vi "ApplicationTemplate.vi"() -> ()   [LabVIEW 2020]
uses:
  VI Server Toolkit/VI Server Toolkit LV2013.lvlib
panel:
  in  "Stop":bool
  out "error out":errorcluster
  in  "error in (no error)":errorcluster
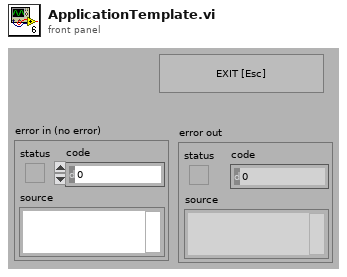
[diagram p1: front panel]
types:
  T1 = typedef "Labels&Control References.ctl" = cluster{"Refs":refnum<vi>[], "Labels":string[], "VI Ref":refnum<vi>}
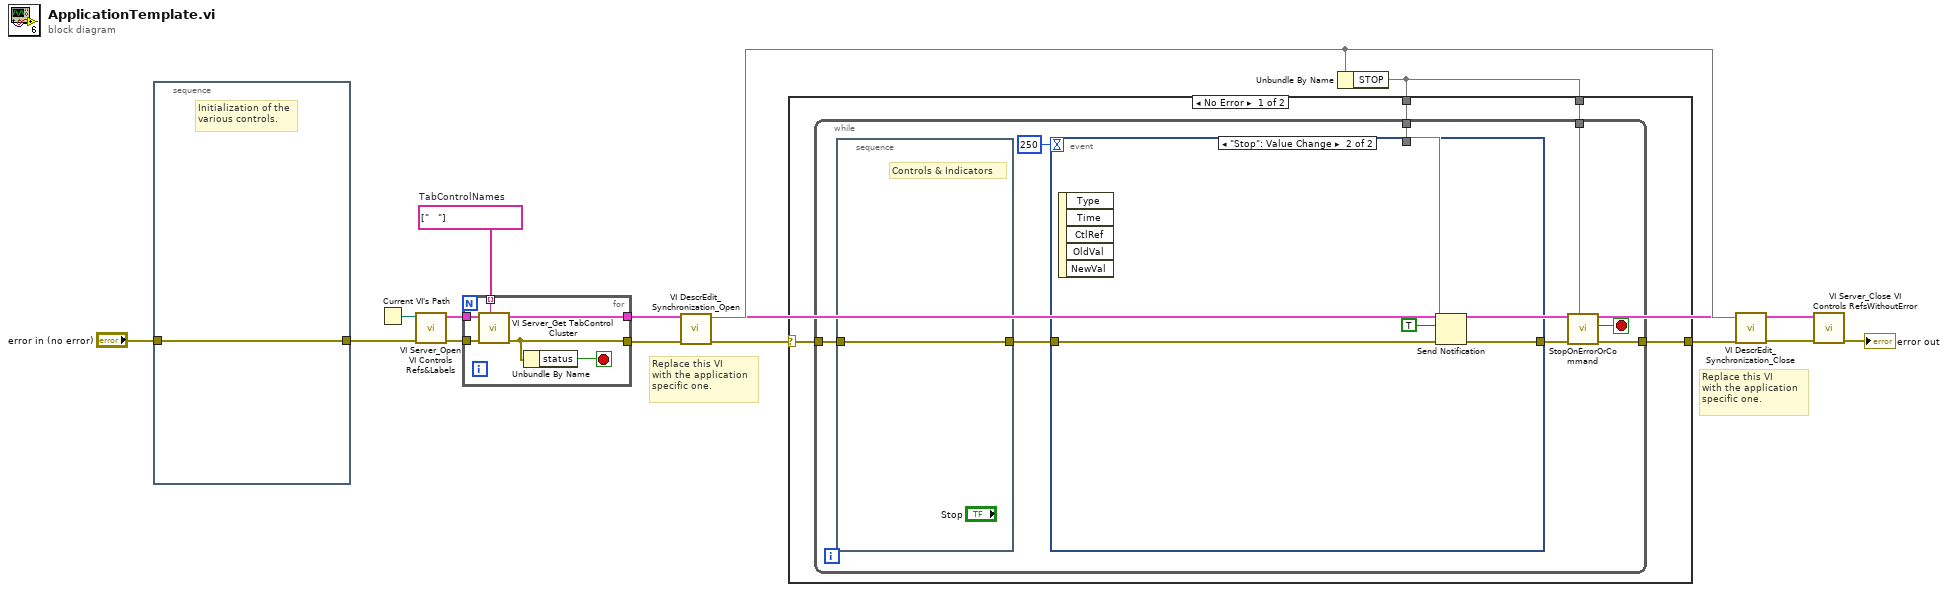
[diagram p0: block diagram]
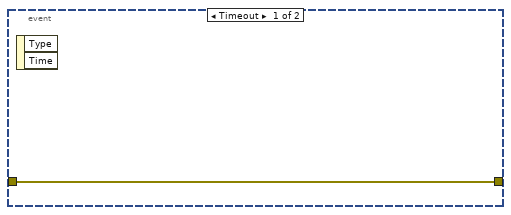
[diagram p2: hidden frame]
diagram:
  w9 = string[] ["   "]  # TabControlNames
  # "Replace this VI\nwith the application\nspecific one."
  # "Replace this VI\nwith the application\nspecific one."
  n1 = stacked-sequence {
    tunnel: "error in (no error)" -> [w15]
    tunnel: [w15] -> w13
    frame #0 {
      # "Initialization of the\nvarious controls."
    }
  }
  n2 = Current VI's Path() -> (path=w12:path)
  n3 = call "VI Server_Open VI Controls Refs&Labels.vi"("error in (no error)"=w13, "vi path"=w12) -> ("error out"=w11:errorcluster, "Labels&Refs"=w10:T1)  [unwired: 8 in]
  n4 = for {
    tunnel: w11 -> [w21]
    tunnel: w10 -> [w20]
    tunnel: [w17] -> w8
    tunnel: [w19] -> w2
    tunnel: w9 -> [w18] mode=indexing
    stop <- w16 stop-if-true
    n5 = call "VI Server_Get TabControl Cluster.vi"("TabControl Label"=w18, "error in"=w21, "VI Server Cluster.IN"=w20) -> ("error out"=w17:errorcluster, "VI Server Cluster.OUT"=w19:T1)  [unwired: 7 in]
    n6 = Unbundle By Name(w17) -> ("status"=w16:bool)
  }
  n7 = call "VI DescrEdit_Synchronization_Open.vi"("error in (no error)"=w8) -> ("error out"=w7:errorcluster, 3:w5)  [unwired: 9 in]
  n8 = Unbundle By Name(w5) -> ("STOP"=w4)
  n9 = case shown="No Error" w7 {
    selector: w7 -> [w25 w40]
    tunnel: [w24 w40] -> w6
    tunnel: w4 -> [w23 _]
    tunnel: w4 -> [w22 _]
    frame No Error {
      n10 = while {
        tunnel: w25 -> [w33]
        tunnel: [w30] -> w24
        tunnel: w23 -> [w28]
        tunnel: w22 -> [w26]
        stop <- w27 stop-if-true
        n11 = stacked-sequence {
          tunnel: w33 -> [w39]
          tunnel: [w39] -> w31
          frame #0 {
            # "Controls & Indicators"
          }
        }
        n12 = event shown="[1] \"Stop\": Value Change" {
          selector: _ -> [_ _]
          dyn-events: _ -> [_ _]
          timeout: 250 -> [_ _]
          tunnel: w31 -> [w34 w38]
          tunnel: [w34 w37] -> w29
          tunnel: w26 -> [_ w36]
          event Timeout {
            n13 = event-data() -> ()  [unwired: 1 in, 2 out]
          }
          event "Stop": Value Change {
            n14 = event-data() -> ()  [unwired: 1 in, 5 out]
            n15 = Send Notification(notification=TRUE, notifier=w36, error in (no error)=w38) -> (error out=w37:errorcluster)  [unwired: 1 out]
          }
        }
        n16 = call "StopOnErrorOrCommand.vi"("STOP"=w28, "error in (no error)"=w29) -> ("error out"=w30:errorcluster, "STOP"=w27:bool)  [unwired: 8 in]
      }
    }
    frame Error {
    }
  }
  n17 = call "VI DescrEdit_Synchronization_Close.vi"("error in (no error)"=w6, 11:w5) -> ("error out"=w3:errorcluster)  [unwired: 9 in]
  n18 = call "VI Server_Close VI Controls RefsWithoutError.vi"("error in (no error)"=w3, "VI Server Cluster"=w2) -> ("error out"=→"error out":errorcluster)  [unwired: 9 in]
